vi "MouseClickEvent.vi"(8 "error in":errorcluster) -> (0 "error out":errorcluster)   [LabVIEW 2015]
uses:
  user32.dll
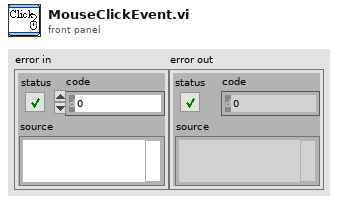
[diagram p1: front panel]
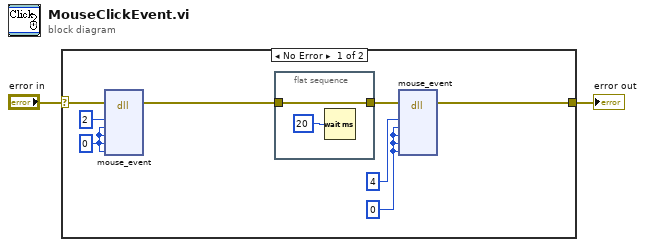
[diagram p0: block diagram]
diagram:
  n1 = case shown="No Error" "error in" {
    selector: "error in" -> [w4 w13]
    tunnel: [w3 w13] -> w1
    frame No Error {
      w7 = 0 ("arg2")
      w8 = 0 ("arg2")
      n2 = dll-call lib="user32.dll" fn="mouse_event"(error in=w4, "arg1"=2, "arg2"=w8, "arg3"=w8, "arg4"=w8, "arg5"=w8) -> (error out=w10:errorcluster)  [unwired: 8 in, 1 out]
      n3 = flat-sequence {
        tunnel: [w11] -> w9
        tunnel: w10 -> [w11]
        frame #0 {
          n4 = Wait (ms)(milliseconds to wait=u32 20) -> ()  [unwired: 1 out]
        }
      }
      n5 = dll-call lib="user32.dll" fn="mouse_event"(error in=w9, "arg1"=4, "arg2"=w7, "arg3"=w7, "arg4"=w7, "arg5"=w7) -> (error out=w3:errorcluster)  [unwired: 8 in, 1 out]
    }
    frame Error {
    }
  }
  "error out" <- w1
